vi "reql_encode.vi"(8 "error in (no error)":errorcluster, 10 "key (\"\")":string, 11 "object":variant) -> (0 "error out":errorcluster, 3 "reql":string)   [LabVIEW 2017, in "rethinkdb.lvlib"]
uses:
  rethinkdb.lvlib
  ql2_term.ctl
  <vilib>/Utility/Data Type/NI_Data Type.lvlib
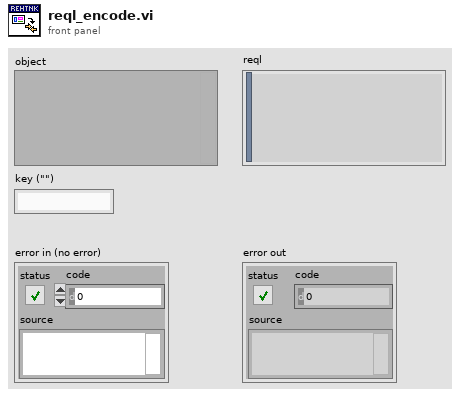
[diagram p1: front panel]
types:
  T1 = typedef "rethinkdb.lvlib/ql2_term.ctl" = enum8{"ADD", "AND", "APPEND", "APRIL", "ARGS", "ASC", "AUGUST", "AVG", "BETWEEN", "BETWEEN_DEPRECATED", "BINARY", "BIT_AND", "BIT_NOT", "BIT_OR", "BIT_SAL", "BIT_SAR", "BIT_XOR", "BRACKET", "BRANCH", "CEIL", "CHANGES", "CHANGE_AT", "CIRCLE", "COERCE_TO", "CONCAT_MAP", "CONFIG", "CONTAINS", "COUNT", "DATE", "DATUM", "DAY", "DAY_OF_WEEK", "DAY_OF_YEAR", "DB", "DB_CREATE", "DB_DROP", "DB_LIST", "DECEMBER", "DEFAULT", "DELETE", "DELETE_AT", "DESC", "DIFFERENCE", "DISTANCE", "DISTINCT", "DIV", "DOWNCASE", "DURING", "EPOCH_TIME", "EQ", "EQ_JOIN", "ERROR", "FEBRUARY", "FILL", "FILTER", "FLOOR", "FOLD", "FOR_EACH", "FRIDAY", "FUNC", "FUNCALL", "GE", "GEOJSON", "GET", "GET_ALL", "GET_FIELD", "GET_INTERSECTING", "GET_NEAREST", "GET_WRITE_HOOK", "GRANT", "GROUP", "GT", "HAS_FIELDS", "HOURS", "HTTP", "IMPLICIT_VAR", "INCLUDES", "INDEX_CREATE", "INDEX_DROP", "INDEX_LIST", "INDEX_RENAME", "INDEX_STATUS", "INDEX_WAIT", "INFO", "INNER_JOIN", "INSERT", "INSERT_AT", "INTERSECTS", "IN_TIMEZONE", "ISO8601", "IS_EMPTY", "JANUARY", "JAVASCRIPT", "JSON", "JULY", "JUNE", "KEYS", "LE", "LIMIT", "LINE", "LITERAL", "LT", "MAKE_ARRAY", "MAKE_OBJ", "MAP", "MARCH", "MATCH", "MAX", "MAXVAL", "MAY", "MERGE", "MIN", "MINUTES", "MINVAL", "MOD", "MONDAY", "MONTH", "MUL", "NE", "NOT", "NOVEMBER", "NOW", "NTH", "OBJECT", "OCTOBER", "OFFSETS_OF", "OR", "ORDER_BY", "OUTER_JOIN", "PLUCK", "POINT", "POLYGON", "POLYGON_SUB", "PREPEND", "RANDOM", "RANGE", "REBALANCE", "RECONFIGURE", "REDUCE", "REPLACE", "ROUND", "SAMPLE", "SATURDAY", "SECONDS", "SEPTEMBER", "SET_DIFFERENCE", "SET_INSERT", "SET_INTERSECTION", "SET_UNION", "SET_WRITE_HOOK", "SKIP", "SLICE", "SPLICE_AT", "SPLIT", "STATUS", "SUB", "SUM", "SUNDAY", "SYNC", "TABLE", "TABLE_CREATE", "TABLE_DROP", "TABLE_LIST", "THURSDAY", "TIME", "TIMEZONE", "TIME_OF_DAY", "TO_EPOCH_TIME", "TO_GEOJSON", "TO_ISO8601", "TO_JSON_STRING", "TUESDAY", "TYPE_OF", "UNGROUP", "UNION", "UPCASE", "UPDATE", "UUID", "VALUES", "VAR", "WAIT", "WEDNESDAY", "WITHOUT", "WITH_FIELDS", "YEAR", "ZIP", "invalid"}
  T2 = typedef "NI_Data Type.lvlib/Data Type.ctl" = enum8{"Invalid Type", "Void", "I8", "I16", "I32", "I64", "U8", "U16", "U32", "U64", "Single Float", "Double Float", "Extended Float", "Single Complex", "Double Complex", "Extended Complex", "Enum U8", "Enum U16", "Enum U32", "Enum U64", "Single Float With Unit", "Double Float With Unit", "Extended Float With Unit", "Single Complex with Unit", "Double Complex with Unit", "Extended Complex with Unit", "Boolean", "String", "Path", "Picture", "Tag", "Array", "Cluster", "Variant", "LV Variant", "Waveform", "Timestamp", "Digital Waveform", "Digital Data", "ExpressData", "Refnum", "External Data", "VI", "Poly VI", "LabVIEW Class Instance", "Fixed Point"}
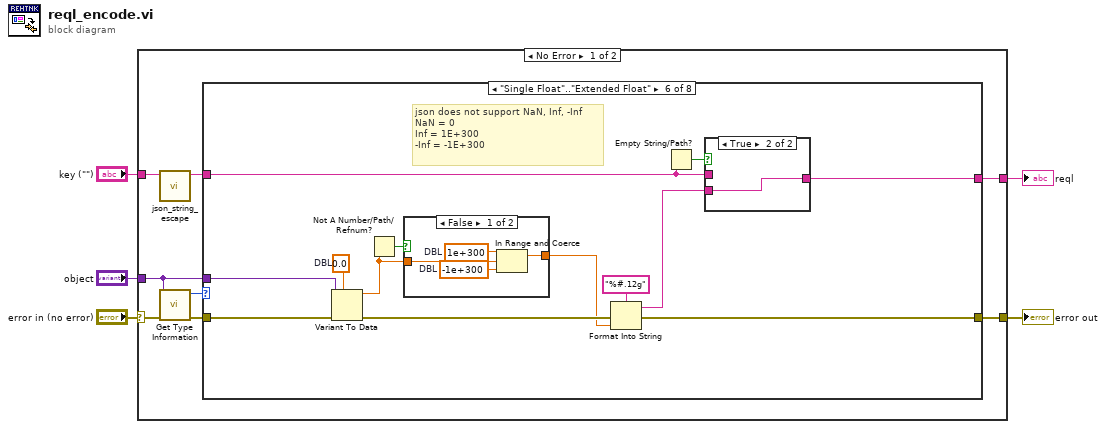
[diagram p0: block diagram]
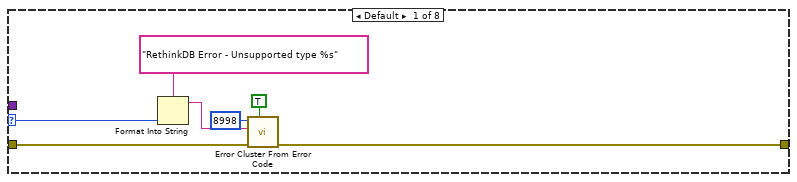
[diagram p2: hidden frame]
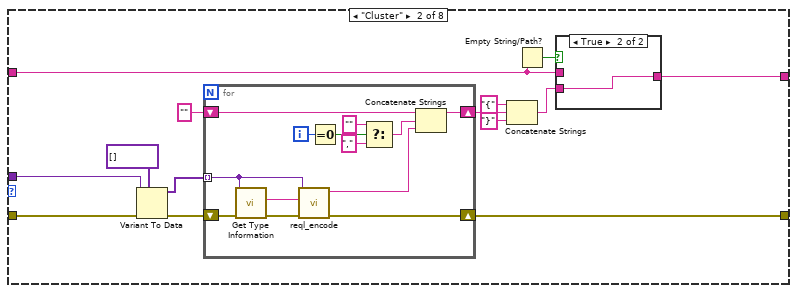
[diagram p3: hidden frame]
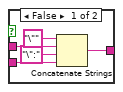
[diagram p4: hidden frame]
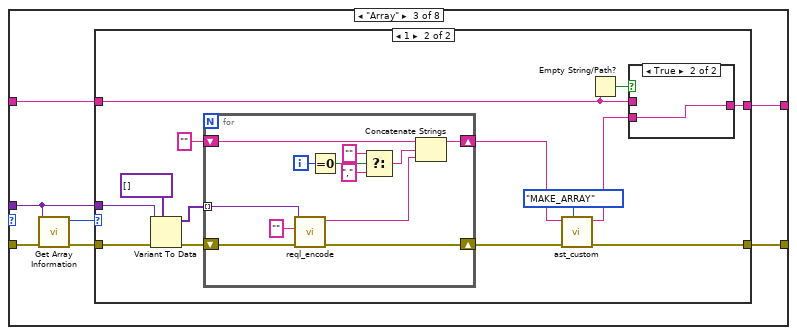
[diagram p5: hidden frame]
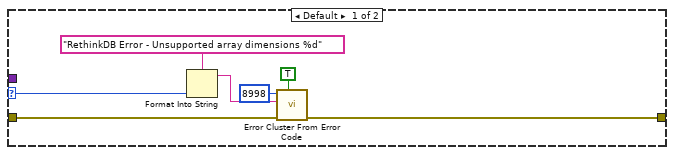
[diagram p6: hidden frame]
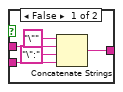
[diagram p7: hidden frame]
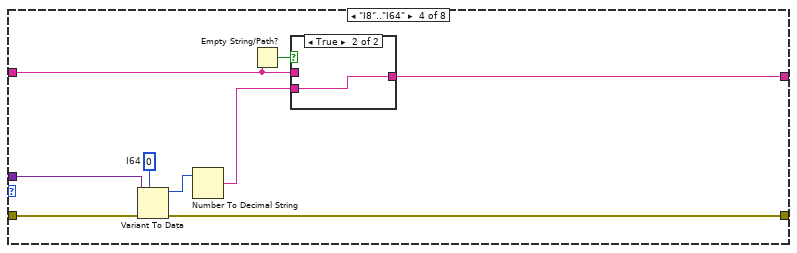
[diagram p8: hidden frame]
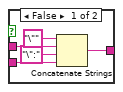
[diagram p9: hidden frame]
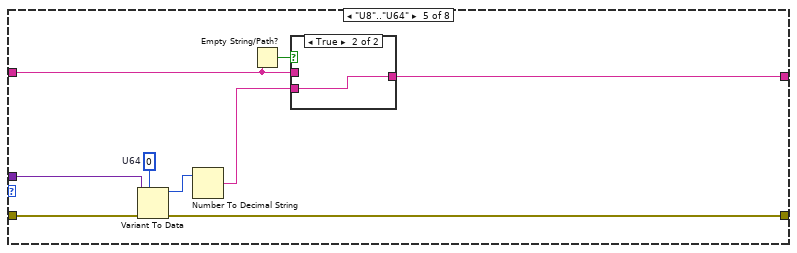
[diagram p10: hidden frame]
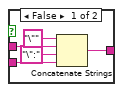
[diagram p11: hidden frame]
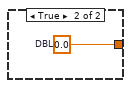
[diagram p12: hidden frame]
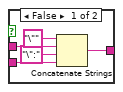
[diagram p13: hidden frame]
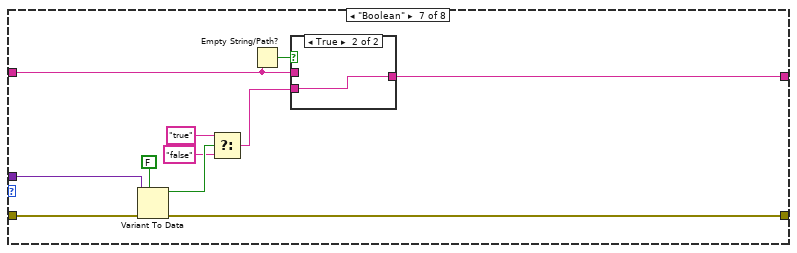
[diagram p14: hidden frame]
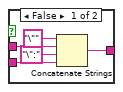
[diagram p15: hidden frame]
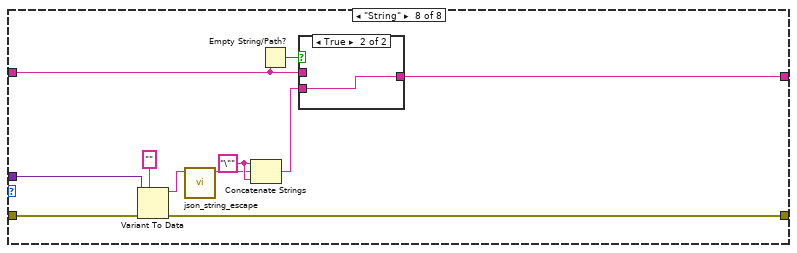
[diagram p16: hidden frame]
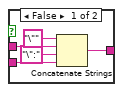
[diagram p17: hidden frame]
diagram:
  n1 = case shown="No Error" "error in (no error)" {
    selector: "error in (no error)" -> [w8 w188]
    tunnel: [w10 w188] -> w5
    tunnel: [w9 _] -> w4
    tunnel: "object" -> [w7 _]
    tunnel: "key (\"\")" -> [w6 _]
    frame No Error {
      n2 = call "json_string_escape.vi"("string"=w6) -> ("escaped string"=w11:string)  [unwired: 10 in]
      n3 = call <vilib>:"Get Type Information.vi"("error in (no error)"=w8, "Variant"=w7) -> ("error out"=w12:errorcluster, "Type"=w13:T2)  [unwired: 5 in, 3 out]
      n4 = case shown="\"Single Float\"..\"Extended Float\"" w13 {
        selector: w13 -> [w16 _ _ _ _ _ _ _]
        tunnel: w7 -> [_ w33 w56 w107 w122 w141 w163 w180]
        tunnel: w12 -> [w20 w34 w57 w108 w123 w142 w164 w181]
        tunnel: [w19 w31 w60 w103 w118 w135 w158 w176] -> w10
        tunnel: [_ w26 w59 w102 w117 w138 w162 w179] -> w9
        tunnel: w11 -> [_ w25 w58 w101 w116 w137 w161 w178]
        frame Default {
          n5 = Format Into String(format string="RethinkDB Error - Unsupported type %s" ("error message (\"\")"), w16) -> (resulting string=w14:string)  [unwired: 2 in, 1 out]
          n6 = call <vilib>:"Error Cluster From Error Code.vi"("show call chain? (False)"=TRUE, "error in (no error)"=w20, "error message (\"\")"=w14, "error code (0)"=8998) -> ("error out"=w19:errorcluster)  [unwired: 5 in]
        }
        frame "Cluster" {
          n7 = Variant To Data(error in=w34, type=variant[] [], Variant=w33) -> (data=w29:variant[], error out=w30:errorcluster)
          n8 = for {
            shift-right: [w44] -> w31
            shift-left: w30 -> [w53]
            tunnel: w29 -> [w42] mode=indexing
            shift-right: [w51] -> w24
            shift-left: "" -> [w52]
            i -> [w50]
            n9 = call <vilib>:"Get Type Information.vi"("error in (no error)"=w53, "Variant"=w42) -> ("error out"=w45:errorcluster, "Name"=w43:string)  [unwired: 5 in, 3 out]
            n10 = call "reql_encode.vi"("error in (no error)"=w45, "key (\"\")"=w43, "object"=w42) -> ("error out"=w44:errorcluster, "reql"=w41:string)  [unwired: 7 in]
            n11 = Equal To 0?(x=w50) -> (x = 0?=w49:bool)
            n12 = Select(t="", s=w49, f="," ("string")) -> (s? t:f=w46:string)
            n13 = Concatenate Strings(w52, w46, w41) -> (w51:string)
          }
          n14 = Concatenate Strings("{" ("string"), w24, "}" ("string")) -> (w23:string)
          n15 = Empty String/Path?(string/path=w25) -> (empty?=w27:bool)
          n16 = case shown="True" w27 {
            tunnel: w23 -> [w37 w40]
            tunnel: [w36 w40] -> w26
            tunnel: w25 -> [w35 _]
            frame False {
              n17 = Concatenate Strings("\"" ("string"), w35, "\":" ("string"), w37) -> (w36:string)
            }
            frame True {
            }
          }
        }
        frame "Array" {
          n18 = call <vilib>:"Get Array Information.vi"("error in (no error)"=w57, "Variant"=w56) -> ("error out"=w55:errorcluster, "Number of Dimensions"=w54:i32)  [unwired: 6 in, 2 out]
          n19 = case shown="1" w54 {
            selector: w54 -> [w62 _]
            tunnel: [w61 w71] -> w60
            tunnel: [_ w76] -> w59
            tunnel: w58 -> [_ w75]
            tunnel: w56 -> [_ w74]
            tunnel: w55 -> [w63 w73]
            frame Default {
              n20 = Format Into String(format string="RethinkDB Error - Unsupported array dimensions %d" ("error message (\"\")"), w62) -> (resulting string=w64:string)  [unwired: 2 in, 1 out]
              n21 = call <vilib>:"Error Cluster From Error Code.vi"("show call chain? (False)"=TRUE, "error in (no error)"=w63, "error message (\"\")"=w64, "error code (0)"=8998) -> ("error out"=w61:errorcluster)  [unwired: 5 in]
            }
            frame 1 {
              n22 = Variant To Data(error in=w73, type=variant[] [], Variant=w74) -> (data=w79:variant[], error out=w80:errorcluster)
              n23 = for {
                shift-right: [w91] -> w72
                shift-left: w80 -> [w92]
                tunnel: w79 -> [w89] mode=indexing
                shift-right: [w98] -> w68
                shift-left: "" -> [w99]
                i -> [w97]
                n24 = call "reql_encode.vi"("error in (no error)"=w92, "key (\"\")"="" ("key"), "object"=w89) -> ("error out"=w91:errorcluster, "reql"=w90:string)  [unwired: 7 in]
                n25 = Equal To 0?(x=w97) -> (x = 0?=w96:bool)
                n26 = Select(t="", s=w96, f="," ("string")) -> (s? t:f=w93:string)
                n27 = Concatenate Strings(w99, w93, w90) -> (w98:string)
              }
              n28 = call "ast_custom.vi"("term_type"=ql2_term."MAKE_ARRAY", "error in (no error)"=w72, "arg0"=w68) -> ("error out"=w71:errorcluster, "r"=w69:string)  [unwired: 7 in]
              n29 = Empty String/Path?(string/path=w75) -> (empty?=w77:bool)
              n30 = case shown="True" w77 {
                tunnel: w69 -> [w84 w87]
                tunnel: [w83 w87] -> w76
                tunnel: w75 -> [w82 _]
                frame False {
                  n31 = Concatenate Strings("\"" ("string"), w82, "\":" ("string"), w84) -> (w83:string)
                }
                frame True {
                }
              }
            }
          }
        }
        frame "I8".."I64" {
          w106 = i64 0  # I64
          n32 = Variant To Data(error in=w108, type=w106, Variant=w107) -> (data=w105:i64, error out=w103:errorcluster)
          n33 = Number To Decimal String(number=w105) -> (decimal integer string=w104:string)  [unwired: 1 in]
          n34 = Empty String/Path?(string/path=w101) -> (empty?=w100:bool)
          n35 = case shown="True" w100 {
            tunnel: w104 -> [w111 w114]
            tunnel: [w110 w114] -> w102
            tunnel: w101 -> [w109 _]
            frame False {
              n36 = Concatenate Strings("\"" ("string"), w109, "\":" ("string"), w111) -> (w110:string)
            }
            frame True {
            }
          }
        }
        frame "U8".."U64" {
          w121 = u64 0  # U64
          n37 = Variant To Data(error in=w123, type=w121, Variant=w122) -> (data=w120:u64, error out=w118:errorcluster)
          n38 = Number To Decimal String(number=w120) -> (decimal integer string=w119:string)  [unwired: 1 in]
          n39 = Empty String/Path?(string/path=w116) -> (empty?=w115:bool)
          n40 = case shown="True" w115 {
            tunnel: w119 -> [w126 w129]
            tunnel: [w125 w129] -> w117
            tunnel: w116 -> [w124 _]
            frame False {
              n41 = Concatenate Strings("\"" ("string"), w124, "\":" ("string"), w126) -> (w125:string)
            }
            frame True {
            }
          }
        }
        frame "Single Float".."Extended Float" {
          w140 = 0.0  # DBL
          # "json does not support NaN, Inf, -Inf\nNaN = 0\nInf = 1E+300\n-Inf = -1E+300"
          n42 = Variant To Data(error in=w142, type=w140, Variant=w141) -> (data=w132:dbl, error out=w139:errorcluster)
          n43 = Not A Number/Path/Refnum?(number/path/refnum=w132) -> (NaN/Path/Refnum?=w131:bool)
          n44 = case shown="False" w131 {
            tunnel: w132 -> [w144 _]
            tunnel: [w143 w147] -> w130
            frame False {
              w145 = 1e+300  # DBL
              w146 = -1e+300  # DBL
              n45 = In Range and Coerce(upper limit=w145, x=w144, lower limit=w146) -> (coerced(x)=w143:dbl)  [unwired: 1 out]
            }
            frame True {
              w147 = 0.0  # DBL
            }
          }
          n46 = Format Into String(format string="%#.12g", error in=w139, w130) -> (resulting string=w133:string, error out=w135:errorcluster)  [unwired: 1 in]
          n47 = Empty String/Path?(string/path=w137) -> (empty?=w136:bool)
          n48 = case shown="True" w136 {
            tunnel: w133 -> [w150 w153]
            tunnel: [w149 w153] -> w138
            tunnel: w137 -> [w148 _]
            frame False {
              n49 = Concatenate Strings("\"" ("string"), w148, "\":" ("string"), w150) -> (w149:string)
            }
            frame True {
            }
          }
        }
        frame "Boolean" {
          n50 = Variant To Data(error in=w164, type=FALSE, Variant=w163) -> (data=w157:bool, error out=w158:errorcluster)
          n51 = Select(t="true", s=w157, f="false") -> (s? t:f=w156:string)
          n52 = Empty String/Path?(string/path=w161) -> (empty?=w160:bool)
          n53 = case shown="True" w160 {
            tunnel: w156 -> [w167 w170]
            tunnel: [w166 w170] -> w162
            tunnel: w161 -> [w165 _]
            frame False {
              n54 = Concatenate Strings("\"" ("string"), w165, "\":" ("string"), w167) -> (w166:string)
            }
            frame True {
            }
          }
        }
        frame "String" {
          w173 = "\"" ("string")
          n55 = Variant To Data(error in=w181, type="", Variant=w180) -> (data=w172:string, error out=w176:errorcluster)
          n56 = call "json_string_escape.vi"("string"=w172) -> ("escaped string"=w171:string)  [unwired: 10 in]
          n57 = Concatenate Strings(w173, w171, w173) -> (w174:string)
          n58 = Empty String/Path?(string/path=w178) -> (empty?=w177:bool)
          n59 = case shown="True" w177 {
            tunnel: w174 -> [w184 w187]
            tunnel: [w183 w187] -> w179
            tunnel: w178 -> [w182 _]
            frame False {
              n60 = Concatenate Strings("\"" ("string"), w182, "\":" ("string"), w184) -> (w183:string)
            }
            frame True {
            }
          }
        }
      }
    }
    frame Error {
    }
  }
  "error out" <- w5
  "reql" <- w4
